vi "PI-C867-SelectVelocity.vi"(8 "error in (no error)":errorcluster, 10 "Velocity array":dbl[](array[numeric]), 11 "State":bool[][](array[boolean])=[[FALSE], [FALSE], [FALSE], [FALSE], [FALSE], [FALSE]]) -> (0 "error out":errorcluster, 3 "Velocity out":dbl)   [LabVIEW 2024]
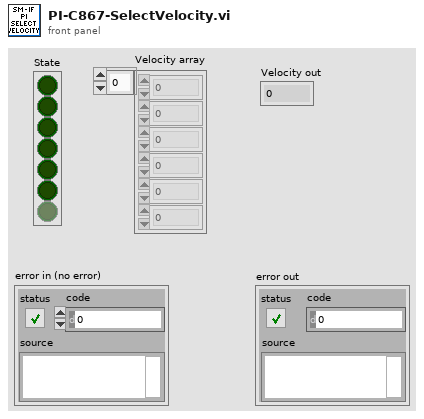
[diagram p1: front panel]
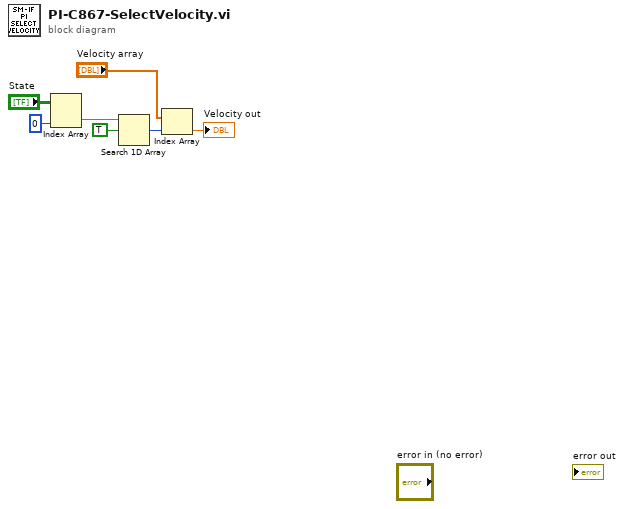
[diagram p0: block diagram]
diagram:
  n1 = Index Array(array="State", index (col)=0 ("disabled index (col)")) -> (element=w5:bool[])  [unwired: 1 in]
  n2 = Search 1D Array(1D array=w5, element=TRUE) -> (index of element=w3:i32)  [unwired: 1 in]
  n3 = Index Array(array="Velocity array", index=w3) -> (element=→"Velocity out":dbl)
